vi "notch core 3.vi"(8 "reset":bool, 9 "coeff":i32, 10 "index":i16, 11 "data in":fxp<+/-,16,1>) -> (1 "output valid!":bool, 3 "data out":fxp<+/-,16,1>)   [LabVIEW 2018, in "SCTL.lvlib"]
uses:
  SCTL.lvlib
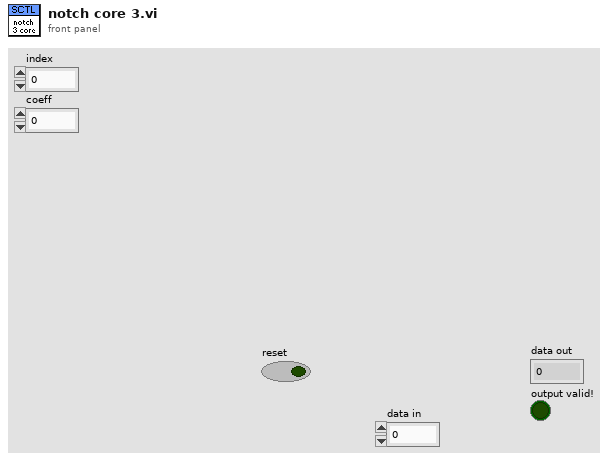
[diagram p1: front panel]
types:
  T1 = cluster{"A*B+C":i32, i32, "filter state in":cluster{"y(n-k)":i32, "x(n-2)":i16, "x(n-1)":i16}}
  T2 = cluster{"y(n-k)":i32, "x(n-2)":i16, "x(n-1)":i16}
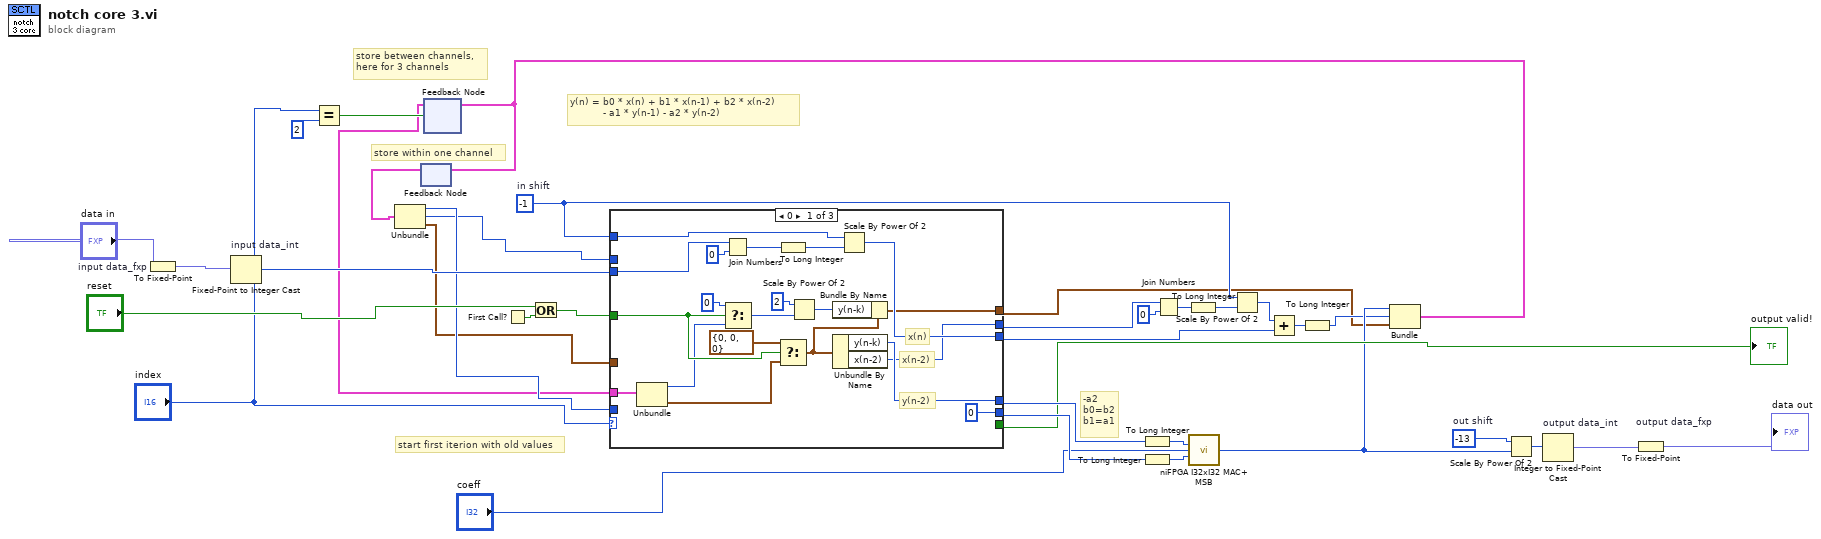
[diagram p0: block diagram]
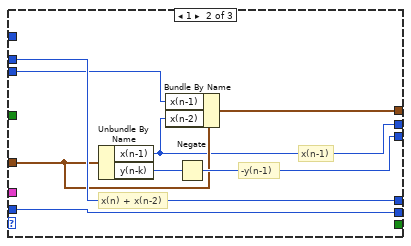
[diagram p2: hidden frame]
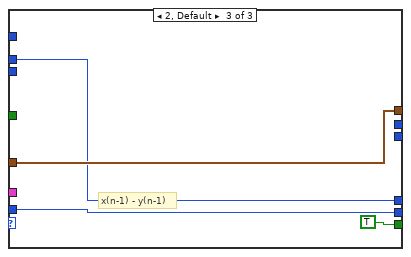
[diagram p3: hidden frame]
diagram:
  w28 = i8 -1  # in shift
  w32 = -13  # out shift
  # "store within one channel"
  # "y(n) = b0 * x(n) + b1 * x(n-1) + b2 * x(n-2)\n           - a1 * y(n-1) - a2 * y(n-2)"
  # "-a2\nb0=b2\nb1=a1"
  # "start first iterion with old values"
  # "store between channels, \nhere for 3 channels"
  n1 = To Fixed-Point "input data_fxp"(number="data in") -> (fixed-point=w36:fxp<+/-,16,1>)  [unwired: 1 out]
  n2 = Fixed-Point to Integer Cast "input data_int"(1:w36) -> (0:w33:i16)
  n3 = Equal?(x="index", y=i16 2) -> (x = y?=w8:bool)
  n4 = feedback #1() -> (w5:T1)  [unwired: 1 in]
  n5 = Unbundle(w5) -> ("A*B+C"=w4:i32, w3:i32, "filter state in"=w2:T2)
  n6 = feedback #2() -> (w1:T1)  [unwired: 1 in]
  n7 = First Call?() -> (First Call?: T/F=w27:bool)
  n8 = Or(x="reset", y=w27) -> (x .or. y?=w31:bool)
  n9 = case shown="0" "index" {
    tunnel: [w41 w59 w68] -> w10
    tunnel: w2 -> [_ w60 w68]
    tunnel: w33 -> [w49 w57 _]
    tunnel: [w53 w62 _] -> w26
    tunnel: w3 -> [_ w63 w66]
    tunnel: [w50 w63 w66] -> w18
    tunnel: [w45 w58 _] -> w20
    tunnel: w4 -> [_ w64 w67]
    tunnel: [0 ("Numeric") w64 w67] -> w24
    tunnel: [_ _ TRUE] -> w13
    tunnel: w31 -> [w44 _ _]
    tunnel: w28 -> [w43 _ _]
    tunnel: w1 -> [w39 _ _]
    frame 0 {
      # "x(n)"
      # "x(n-2)"
      # "y(n-2)"
      n10 = Unbundle(w39) -> ("A*B+C"=w37:i32, "filter state in"=w38:T2)  [unwired: 1 out]
      n11 = Join Numbers(hi=w49, lo=i16 0) -> ((hi.lo)=w56:u32)
      n12 = Select(t=0, s=w44, f=w37) -> (s? t:f=w47:i32)
      n13 = To Long Integer(number=w56) -> (32bit integer=w54:i32)
      n14 = Select(t=T2 {"y(n-k)"=0, "x(n-2)"=0, "x(n-1)"=0} ("filter state in"), s=w44, f=w38) -> (s? t:f=w40:T2)
      n15 = Scale By Power Of 2(n=2, x=w47) -> (x*2^n=w46:i32)
      n16 = Bundle By Name(cluster=w40, "y(n-k)"=w46) -> (w41:T2)
      n17 = Unbundle By Name(w40) -> ("y(n-k)"=w50:i32, "x(n-2)"=w45:i16)
      n18 = Scale By Power Of 2(n=w43, x=w54) -> (x*2^n=w53:i32)
    }
    frame 1 {
      # "x(n) + x(n-2)"
      # "-y(n-1)"
      # "x(n-1)"
      n19 = Unbundle By Name(w60) -> ("x(n-1)"=w58:i16, "y(n-k)"=w61:i32)
      n20 = Bundle By Name(cluster=w60, "x(n-1)"=w57, "x(n-2)"=w58) -> (w59:T2)
      n21 = Negate(x=w61) -> (-x=w62:i32)
    }
    frame 2, Default {
      # "x(n-1) - y(n-1)"
    }
  }
  "output valid!" <- w13
  n22 = To Long Integer(number=w18) -> (32bit integer=w29:i32)
  n23 = To Long Integer(number=w24) -> (32bit integer=w30:i32)
  n24 = Join Numbers(hi=w20, lo=i16 0) -> ((hi.lo)=w21:u32)
  n25 = To Long Integer(number=w21) -> (32bit integer=w22:i32)
  n26 = call <vilib>:"niFPGA I32xI32 MAC+ MSB.vi"("A"=w29, "B"="coeff", "C"=w30) -> ("A*B+C"=w12:i32)  [unwired: 12 in]
  n27 = Scale By Power Of 2(n=w28, x=w22) -> (x*2^n=w19:i32)
  n28 = Add(x=w19, y=w26) -> (x+y=w25:i32)
  n29 = To Long Integer(number=w25) -> (32bit integer=w11:i32)
  n30 = Bundle("A*B+C"=w12, w11, "filter state in"=w10) -> (w6:T1)  [unwired: 1 in]
  n31 = feedback-in #1(w6) -> ()
  n32 = feedback-in #2(w6, w8) -> ()
  n33 = Scale By Power Of 2(n=w32, x=w12) -> (x*2^n=w34:i32)
  n34 = Integer to Fixed-Point Cast "output data_int"(integer=w34) -> (fixed-point=w35:fxp<+/-,32,17>)  [unwired: 1 in]
  n35 = To Fixed-Point "output data_fxp"(number=w35) -> (fixed-point=→"data out":fxp<+/-,16,1>)  [unwired: 1 out]
